vi "crop.vi"(0 "Image in":T1, 1 "left":i32, 2 "right":i32, 3 "top":i32, 4 "bottom":i32, 5 "error in (no error)":errorcluster) -> (14 "Image out":T1, 19 "error out":errorcluster)   [LabVIEW 2022 SP3, in "Vision.lvlib"]
uses:
  Vision.lvlib
  <vilib>/vision/Image Controls.llb/IMAQ Image.ctl
  bin/Vision.dll
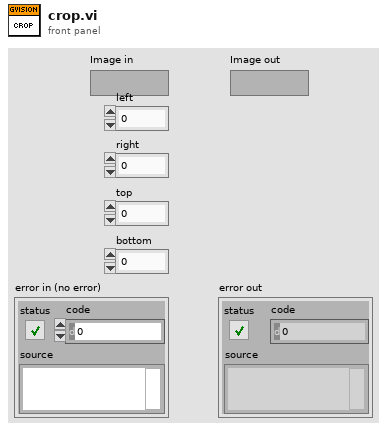
[diagram p1: front panel]
types:
  T1 = typedef "IMAQ Image.ctl" = refnum<image>
  T2 = enum32{"Map Pixel Pointer", "Unmap Pixel Pointer", "Get Pixels Infos"}
  T3 = typedef "Image Type" = u32
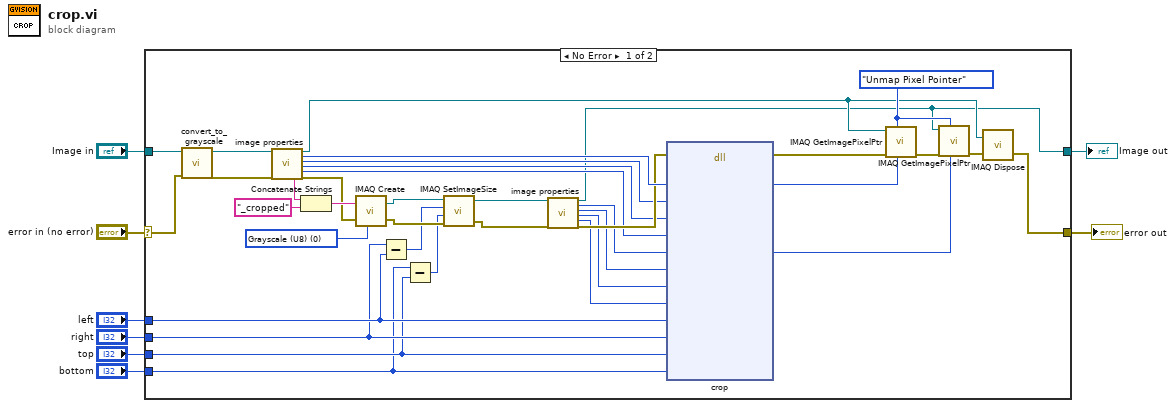
[diagram p0: block diagram]
diagram:
  n1 = case shown="No Error" "error in (no error)" {
    selector: "error in (no error)" -> [w36 w47]
    tunnel: "Image in" -> [w37 w46]
    tunnel: [w45 w47] -> w6
    tunnel: [w9 w46] -> w5
    tunnel: "left" -> [w16 _]
    tunnel: "right" -> [w15 _]
    tunnel: "top" -> [w14 _]
    tunnel: "bottom" -> [w13 _]
    frame No Error {
      w38 = T2."Unmap Pixel Pointer" ("Function")
      w42 = T3 0 items=["Grayscale (U8)", "Grayscale (I16)", "Grayscale (SGL)", "Complex (CSG)", "RGB (U32)", "HSL (U32)", "RGB (U64)", "Grayscale (U16)"] ("Image Type")
      n2 = call "convert_to_grayscale.vi"("error in (no error)"=w36, "Image in"=w37) -> ("error out"=w34:errorcluster, "Image out"=w35:T1)  [unwired: 8 in]
      n3 = call "image properties.vi"("Image in"=w35, "error in (no error)"=w34) -> ("Image Name"=w33:string, "Image out"=w10:T1, "Pixel Pointer out"=w25:u64, "Line Width"=w23:i32, "X Resolution"=w22:i32, "Y Resolution"=w21:i32, "error out"=w31:errorcluster)  [unwired: 11 in]
      n4 = Concatenate Strings(w33, "_cropped" ("string")) -> (w43:string)
      n5 = call "IMAQ Create"("Image Name"=w43, "Image Type"=w42, "error in (no error)"=w31) -> ("New Image"=w32:T1, "error out"=w30:errorcluster)  [unwired: 2 in]
      n6 = Subtract(x=w15, y=w16) -> (x-y=w29:i32)
      n7 = Subtract(x=w13, y=w14) -> (x-y=w28:i32)
      n8 = call "IMAQ SetImageSize"("error in (no error)"=w30, "Y Resolution"=w28, "X Resolution"=w29, "Image"=w32) -> ("error out"=w26:errorcluster, "Image Out"=w27:T1)  [unwired: 1 in]
      n9 = call "image properties.vi"("Image in"=w27, "error in (no error)"=w26) -> ("Image out"=w9:T1, "Pixel Pointer out"=w20:u64, "Line Width"=w19:i32, "X Resolution"=w18:i32, "Y Resolution"=w17:i32, "error out"=w24:errorcluster)  [unwired: 11 in, 1 out]
      n10 = dll-call lib="C:/Users/Caleb/Desktop/nebraska-silicon-lab/pixel-gantry-control/Gantry/Shared Components/External/bin/Vision.dll" fn="crop"(error in=w24, "src_imgPtr"=w25, "src_imgLineWidth"=w23, "src_imgWidth"=w22, "src_imgHeight"=w21, "dst_imgPtr"=w20, "dst_imgLineWidth"=w19, "dst_imgWidth"=w18, "dst_imgHeight"=w17, "left"=w16, "right"=w15, "top"=w14, "bottom"=w13) -> (error out=w40:errorcluster, "src_imgPtr"=w12:u64, "dst_imgPtr"=w11:u64)  [unwired: 13 in, 1 out]
      n11 = call "IMAQ GetImagePixelPtr"("Pixel Pointer in"=w12, "Function"=w38, "error in (no error)"=w40, "Image"=w10) -> ("error out"=w41:errorcluster)  [unwired: 2 in, 5 out]
      n12 = call "IMAQ GetImagePixelPtr"("Pixel Pointer in"=w11, "Function"=w38, "error in (no error)"=w41, "Image"=w9) -> ("error out"=w39:errorcluster)  [unwired: 2 in, 5 out]
      n13 = call "IMAQ Dispose"("Image"=w10, "error in (no error)"=w39) -> ("error out"=w45:errorcluster)  [unwired: 4 in]
    }
    frame Error {
    }
  }
  "Image out" <- w5
  "error out" <- w6
